vi "Outline UPH and cycTime.vi"(8 "error in (no error)":errorcluster, 10 "Model":string, 11 "Cluster":T2) -> (0 "error out":errorcluster, 3 "UPH":dbl)   [LabVIEW 2014]
uses:
  Type'def/FTT Display Type.ctl
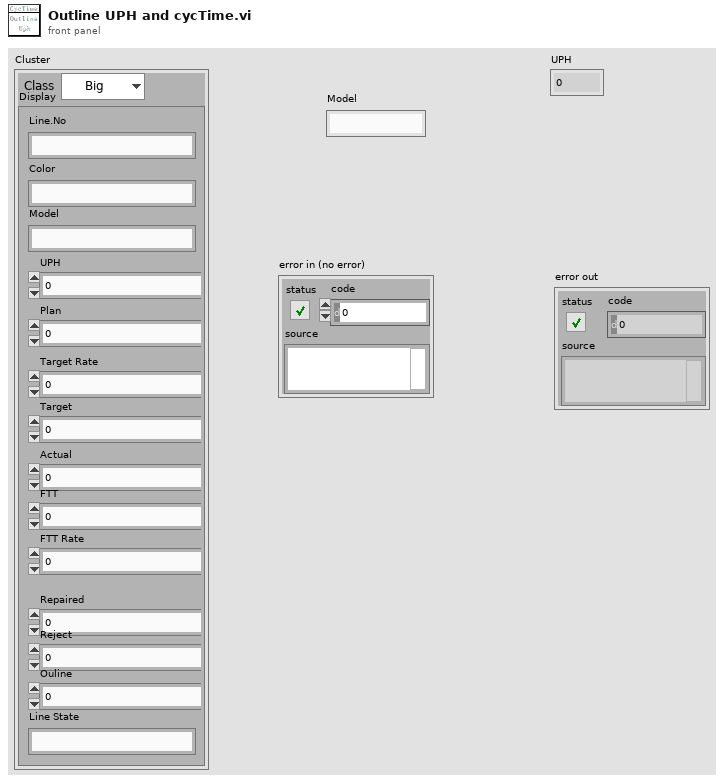
[diagram p1: front panel]
types:
  T1 = typedef "FTT Display Type.ctl" = cluster{"Line.No":string, "Model":string, "Color":string, "UPH":dbl, "Plan":dbl, "Target Rate":dbl, "Target ":dbl, "Actual":dbl, "FTT":dbl, "FTT Rate":dbl, "Repaired":dbl, "Reject":dbl, "Ouline":dbl, "Line State":string}
  T2 = cluster{"Display":T1, "Class":enum16{"Big", "Small"}}
  T3 = typedef "UPH Config.ctl" = cluster{"Line_No":string, "Model":string, "B_UPH ":i16, "S_UPH  ":i16, "Class":enum16{"Big", "Small"}}
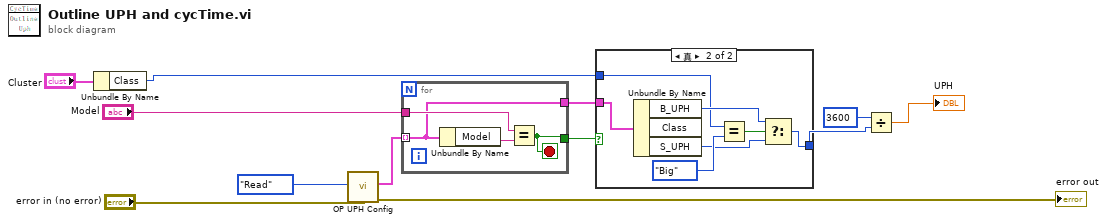
[diagram p0: block diagram]
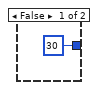
[diagram p2: hidden frame]
diagram:
  n1 = Unbundle By Name("Cluster") -> ("Class"=w7:enum16{"Big", "Small"})
  n2 = call "OP UPH Config.vi"("error in (no error)"="error in (no error)", "Enum"=enum16{"init", "Read", "Write"}."Read") -> ("error out"=→"error out":errorcluster, "UPH out"=w6:T3[])  [unwired: 7 in, 1 out]
  n3 = for {
    tunnel: w6 -> [w14] mode=indexing
    tunnel: "Model" -> [w15]
    tunnel: [w14] -> w4
    tunnel: [w13] -> w5
    stop <- w13 stop-if-true
    n4 = Unbundle By Name(w14) -> ("Model"=w16:string)
    n5 = Equal?(x=w15, y=w16) -> (x = y?=w13:bool)
  }
  n6 = case shown="真" w5 {
    tunnel: w4 -> [_ w24]
    tunnel: [i16 30 ("S_UPH") w19] -> w3
    tunnel: w7 -> [_ w18]
    frame False {
    }
    frame True {
      n7 = Unbundle By Name(w24) -> ("B_UPH"=w21:i16, "S_UPH"=w20:i16)  [unwired: 1 out]
      n8 = Equal?(x=w18, y=enum16{"Big", "Small"}."Big" ("Class")) -> (x = y?=w22:bool)
      n9 = Select(t=w21, s=w22, f=w20) -> (s? t:f=w19:i16)
    }
  }
  n10 = Divide(x=i16 3600, y=w3) -> (x/y=→"UPH":dbl)
